vi "Convert to Double.vi"(8 "error in":errorcluster, 11 "In":i32) -> (0 "error out":errorcluster, 3 "Out":dbl)   [LabVIEW 2026, in "Runtime Configuration Support Example Engine.lvlib"]
uses:
  Runtime Configuration Support Example Engine.lvlib
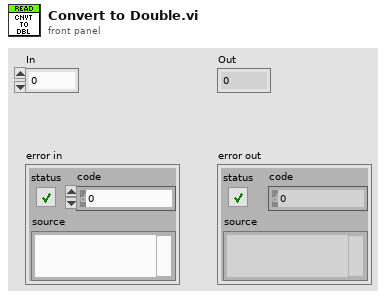
[diagram p1: front panel]
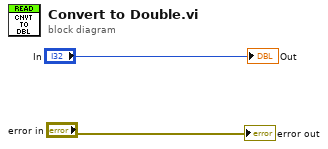
[diagram p0: block diagram]
diagram:
  "Out" <- "In"
  "error out" <- "error in"
